vi "Read error string index.vi"(8 "error in (no error)":errorcluster caption="에러 입력(에러 없음)", 11 "Script Line 입력":refnum<class "Script Line.lvclass">) -> (0 "error out":errorcluster caption="에러 출력", 2 "error string index":cluster{"start":u32, "end":u32}[](array[cluster]), 3 "Script Line 출력":refnum<class "Script Line.lvclass">)   [LabVIEW 2020, in "Script Line.lvclass"]
uses:
  Script Line.lvclass
  Script Line.lvclass/Script Line.ctl
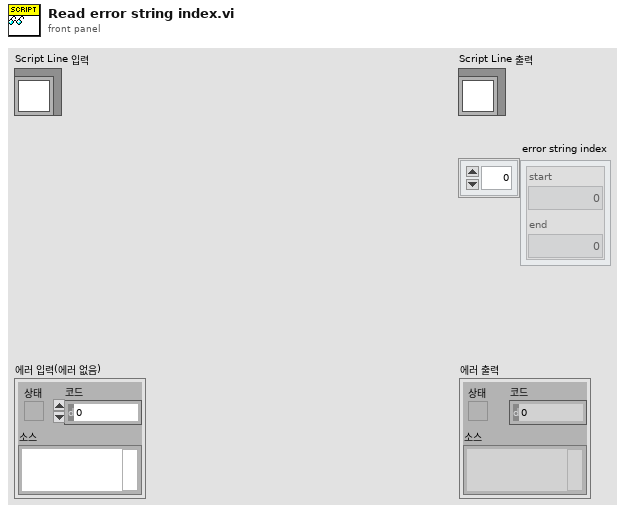
[diagram p1: front panel]
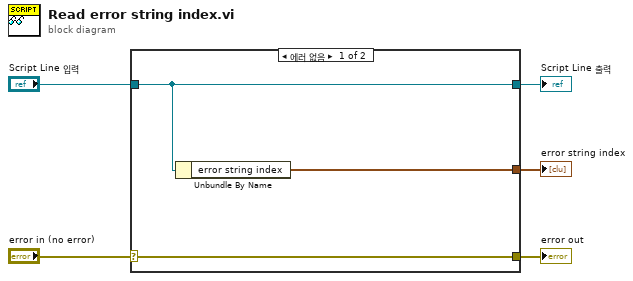
[diagram p0: block diagram]
diagram:
  n1 = case shown="에러 없음" "error in (no error)" {
    selector: "error in (no error)" -> [w8 w9]
    tunnel: [w8 w9] -> w4
    tunnel: [w7 w10] -> w2
    tunnel: "Script Line 입력" -> [w7 w10]
    tunnel: [w6 _] -> w1
    frame No Error {
      n2 = Unbundle By Name(w7) -> ("error string index"=w6:cluster{"start":u32, "end":u32}[])
    }
    frame Error {
    }
  }
  "error out" <- w4
  "Script Line 출력" <- w2
  "error string index" <- w1
